vi "Error Message.vi"(8 "error in (no error)":errorcluster, 10 "Type of Dialog (1: OK Message)":i32(ring)=1 items=["No Dialog", "OK Message", "Continue or Stop Message"], 11 "VISA resource name":refnum<visa-resource-name>) -> (0 "error out":errorcluster, 1 "error message":string, 2 "error code":i32, 3 "VISA resource name out":refnum<visa-resource-name>, 4 "Status":bool)   [LabVIEW 2020, in "Rohde&Schwarz CMXP GPRF.lvlib"]
doc: "This VI takes the status code in its input error cluster and converts it into a user-readable string. You can display the message in a popup-window or just use it as string value."
uses:
  <instrlib>/Rohde&Schwarz CMXP GPRF/Rohde&Schwarz CMXP GPRF.lvlib
  <instrlib>/Rohde&Schwarz CMXP GPRF/Private/rsidr_core.llb/rsidr_core.lvlib
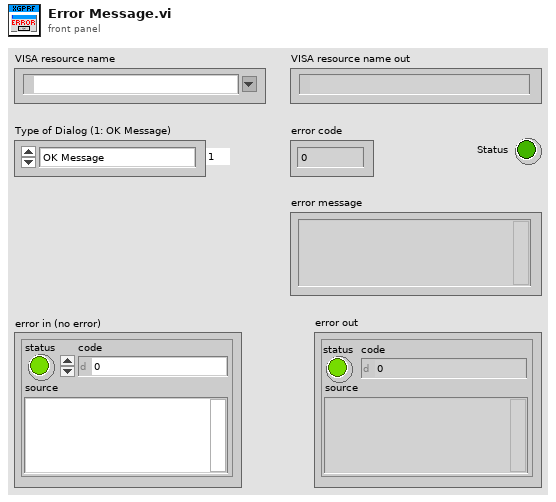
[diagram p1: front panel]
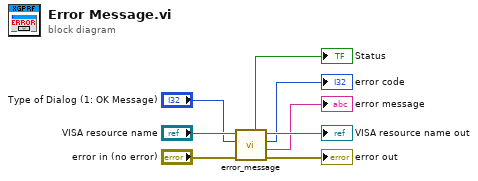
[diagram p0: block diagram]
diagram:
  n1 = call <instrlib>:"error_message.vi"("error in"="error in (no error)", "Type of Dialog (OK Message)"="Type of Dialog (1: OK Message)", "VISA resource name"="VISA resource name") -> ("error out"=→"error out":errorcluster, "error message"=→"error message":string, "error code"=→"error code":i32, "VISA resource name out"=→"VISA resource name out":refnum<visa-resource-name>, "Status"=→"Status":bool)  [unwired: 4 in]
